vi "Resolve Symbolic Path.vi"(1 "Symbolic Path Enum":T1(ring), 2 "Symbolic Path":string) -> (0 "ActualPath":path)   [LabVIEW 2017]
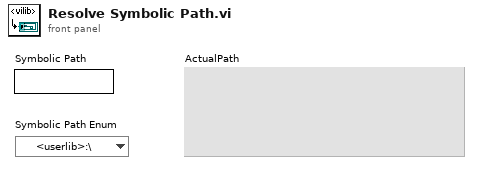
[diagram p1: front panel]
types:
  T1 = enum16{"<userlib>:\\", "<vilib>:\\", "<instrlib>:\\", "<osdatadir>:\\"}
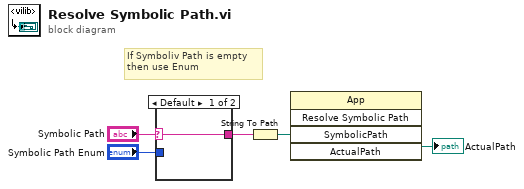
[diagram p0: block diagram]
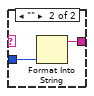
[diagram p2: hidden frame]
diagram:
  # "If Symboliv Path is empty\nthen use Enum"
  n1 = case shown="Default" "Symbolic Path" {
    selector: "Symbolic Path" -> [w6 _]
    tunnel: "Symbolic Path Enum" -> [_ w8]
    tunnel: [w6 w7] -> w3
    frame Default {
    }
    frame "" {
      n2 = Format Into String(w8) -> (resulting string=w7:string)  [unwired: 3 in, 1 out]
    }
  }
  n3 = String To Path(string=w3) -> (path=w2:path)
  n4 = invoke class="App" method="Resolve Symbolic Path"("SymbolicPath"=w2) -> ("ActualPath"=→"ActualPath":path)  [unwired: 4 in, 4 out]
